vi "AllocU64BufferGen.vi"(11 "BuffLength":i32) -> (3 "Buffer":u64[](array[numeric]))   [LabVIEW 2019]
panel:
  out "sortie d'erreur":errorcluster caption="ErrorOut"
  in  "entrée d'erreur":errorcluster caption="ErrorIn"
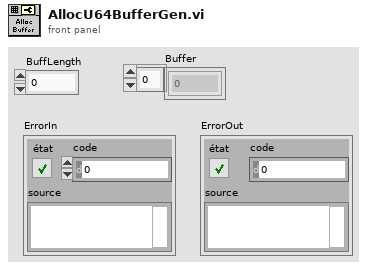
[diagram p1: front panel]
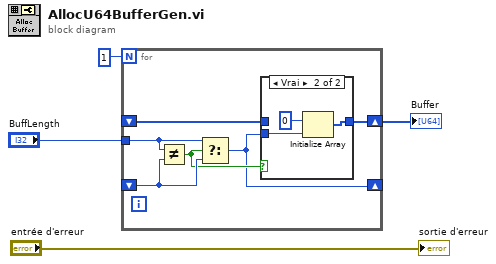
[diagram p0: block diagram]
diagram:
  n1 = for {
    N: 1 -> [_]
    shift-right: [w7] -> _
    shift-left: _ -> [w9]
    tunnel: "BuffLength" -> [w10]
    shift-right: [w6] -> w4
    shift-left: _ -> [w5]
    n2 = Not Equal?(x=w10, y=w9) -> (x != y?=w8:bool)
    n3 = Select(t=w10, s=w8, f=w9) -> (s? t:f=w7:i32)
    n4 = case shown="Vrai" w8 {
      tunnel: w7 -> [_ w14]
      tunnel: [w11 w12] -> w6
      tunnel: w5 -> [w11 _]
      frame False {
      }
      frame True {
        n5 = Initialize Array(u64 0, w14) -> (w12:u64[])
      }
    }
  }
  "Buffer" <- w4
  "sortie d'erreur" <- "entrée d'erreur"
